vi "Application Status View.vi"(0 "Model in":refnum<class "Model.lvclass">) -> ()   [LabVIEW 2016, in "M1M3SupportEUI_Views.lvlib"]
uses:
  M1M3SupportEUI_Views.lvlib
  Model/Model.lvclass
  M1M3 Support Events/M1M3 Support Events.lvclass/M1M3 Support Events.ctl
  M1M3 Support Events/M1M3 Support Events.lvclass
panel:
  out "Force Magnitude":sgl format="%_8f"
  out "Mx":sgl format="%_8f"
  out "My":sgl format="%_8f"
  out "Mz":sgl format="%_8f"
  out "Fz":sgl format="%_8f"
  out "Fy":sgl format="%_8f"
  out "Fx":sgl format="%_8f"
  out "FA Force Warning Status":string
  out "FA Warning Status":string
  out "Summary State":string
  out "Interlock Status":string
  out "Detailed State":string
  # "Applied Forces Event Data"
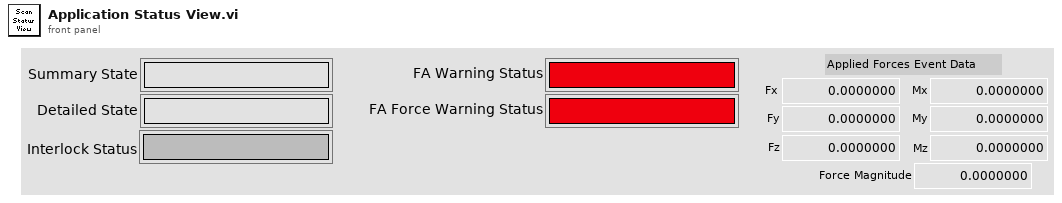
[diagram p1: front panel]
types:
  T1 = typedef "M1M3SupportEUI_TypeDefs.lvlib/M1M3 Support Events.ctl" = cluster{"Inclinometer  Data":refnum<user-event>, "IMS Data":refnum<user-event>, "SAL Connected":refnum<user-event>, "Accelerometer Data":refnum<user-event>, "OuterLoop Data":refnum<user-event>, "ErrorCode Event":refnum<user-event>, "InterlockStatus Event":refnum<user-event>, "InterlockWarning Event":refnum<user-event>, "Gyro Data":refnum<user-event>, "HP Actuator Info Event":refnum<user-event>, " FA Info Event":refnum<user-event>, "HP Monitor Info Event":refnum<user-event>, "FA Data":refnum<user-event>, "HP Actuator data":refnum<user-event>, "HP Monitor data":refnum<user-event>, "Air Supply Status Event":refnum<user-event>, "Air Supply Warning Event":refnum<user-event>, "Power Data":refnum<user-event>, "PID Data":refnum<user-event>, "PID Info Event":refnum<user-event>, "Power Status Event":refnum<user-event>, "Power Supply Status Event":refnum<user-event>, "Power Warning Event":refnum<user-event>, "Summary State Event":refnum<user-event>, "Detailed State Event":refnum<user-event>, "FA Force Warning Event":refnum<user-event>, "FA Warning Event":refnum<user-event>, "FA State Event":refnum<user-event>, "Applied AberrationForces Event":refnum<user-event>, "Applied Acceleration Forcces Event":refnum<user-event>, "Applied Azimuth Forces Event":refnum<user-event>, "Applied Active Optic Forces Event":refnum<user-event>, "Applied Balance Forces Event":refnum<user-event>, "Applied Cylinder Forces Event":refnum<user-event>, "Applied Elevation Forces Event":refnum<user-event>, "Applied Forces Event":refnum<user-event>, "Applied Offset Forces Event":refnum<user-event>, "Applied Static Forces Event":refnum<user-event>, "Applied Thermal Forces Event":refnum<user-event>, "Applied Velocity Forces Event":refnum<user-event>, "Rejected Aberration Force Event":refnum<user-event>, "Rejected Acceleration Forces Event":refnum<user-event>, "Rejected Active Optic Forces Event":refnum<user-event>, "Rejected Azimuth Forces Event":refnum<user-event>, "Rejected Balance Forces Event":refnum<user-event>, "Rejected Cylinder Forces Event":refnum<user-event>, "Rejected Elevation Forces Event":refnum<user-event>, "Rejected Forces Event":refnum<user-event>, "Rejected Offset Forces Event":refnum<user-event>, "Rejected Static Forces Event":refnum<user-event>, "Rejected Thermal Forces Event":refnum<user-event>, "Rejected Velocity Forces Event":refnum<user-event>, "Command Rejection Event":refnum<user-event>, "Setting Verions Event":refnum<user-event>, "Settings Applied Event":refnum<user-event>}
  T2 = enum16{"", "DetailedState_DetailedStates_DisabledState", "DetailedState_DetailedStates_EnabledState", "DetailedState_DetailedStates_FaultState", "DetailedState_DetailedStates_OfflineState", "DetailedState_DetailedStates_StandbyState", "DetailedState_DetailedStates_ParkedState", "DetailedState_DetailedStates_RaisingState", "DetailedState_DetailedStates_ActiveState", "DetailedState_DetailedStates_LoweringState", "DetailedState_DetailedStates_EngineeringState", "DetailedState_DetailedStates_ParkedEngineeringState", "DetailedState_DetailedStates_RaisingEngineeringState", "DetailedState_DetailedStates_ActiveEngineeringState", "DetailedState_DetailedStates_LoweringEngineeringState", "DetailedState_DetailedStates_LoweringFaultState", "DetailedState_DetailedStates_ProfileHardpointCorrectionState"}
  T3 = enum16{"", "SummaryState_SummaryStates_DisabledState", "SummaryState_SummaryStates_EnabledState", "SummaryState_SummaryStates_FaultState", "SummaryState_SummaryStates_OfflineState", "SummaryState_SummaryStates_StandbyState"}
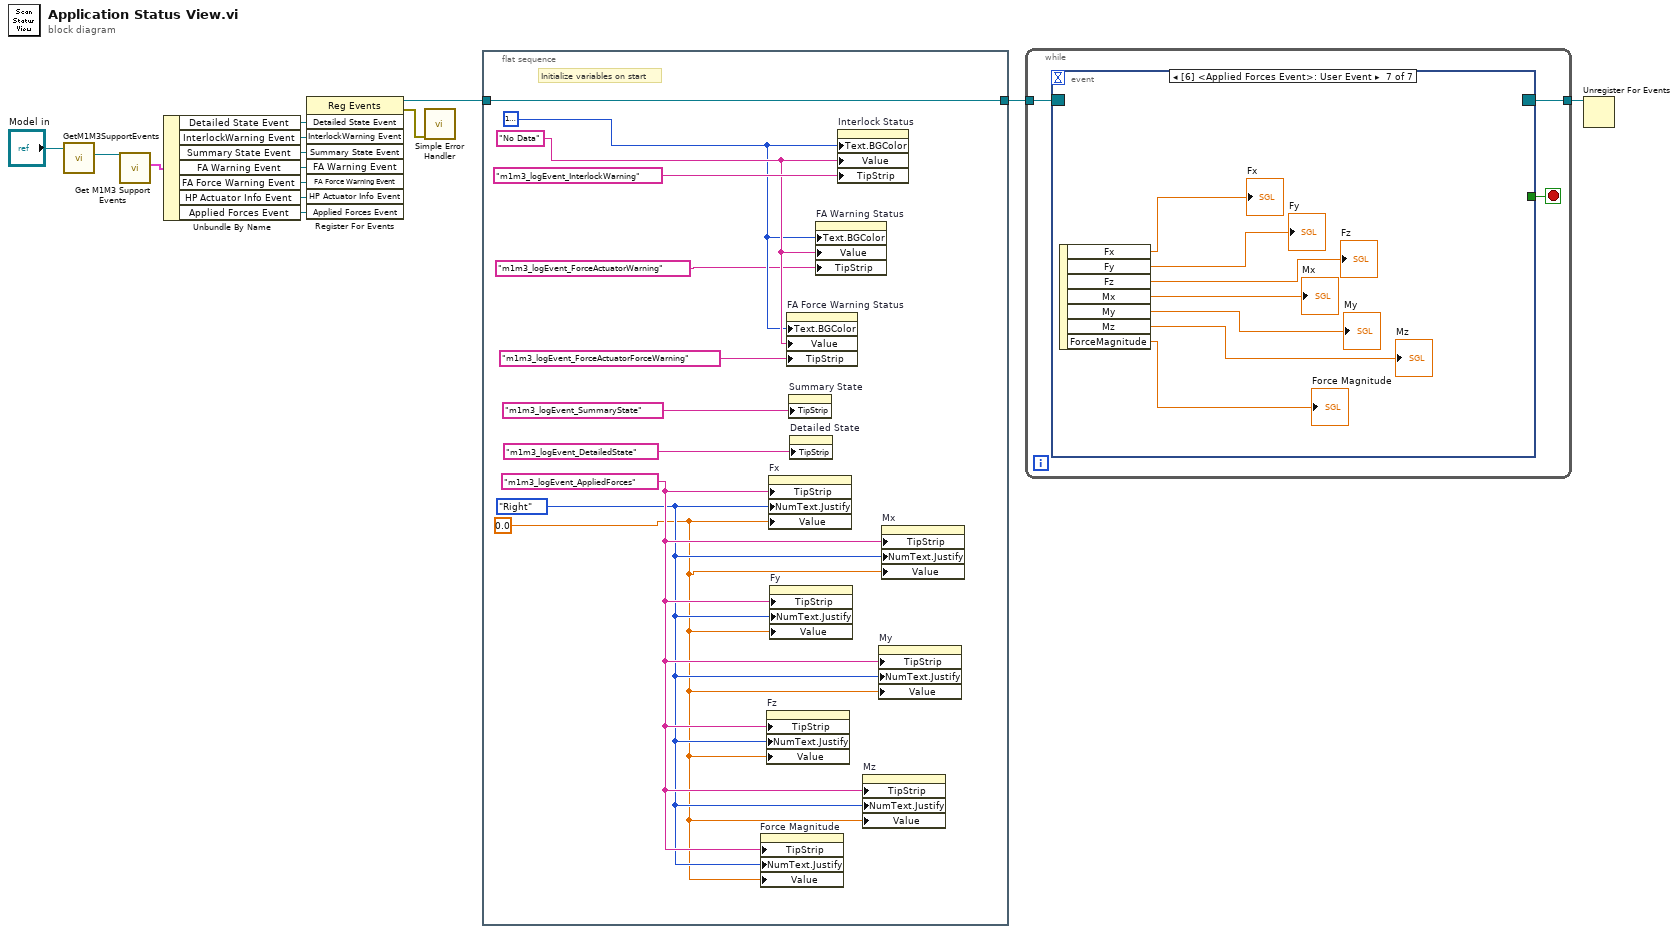
[diagram p0: block diagram]
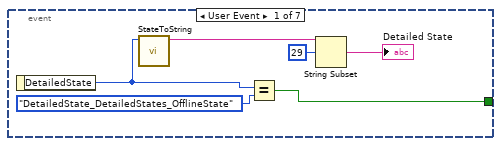
[diagram p2: hidden frame]
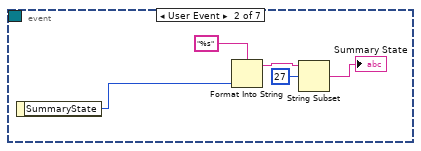
[diagram p3: hidden frame]
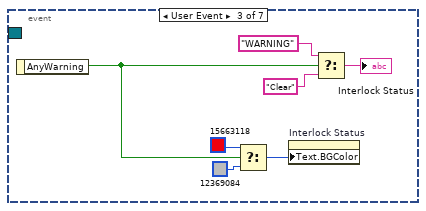
[diagram p4: hidden frame]
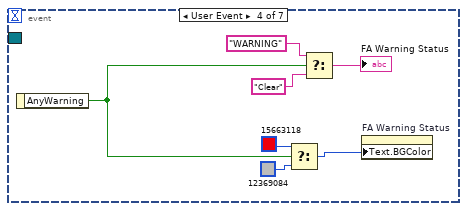
[diagram p5: hidden frame]
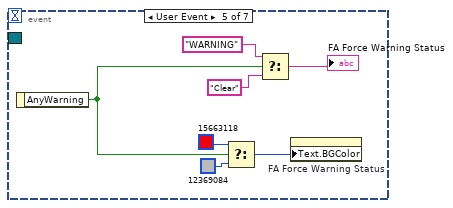
[diagram p6: hidden frame]
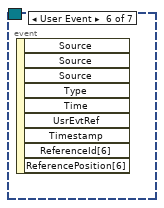
[diagram p7: hidden frame]
diagram:
  n1 = call "GetM1M3SupportEvents.vi"("Model in"="Model in") -> ("M1M3 Support Events out"=w9:refnum<class "M1M3 Support Events.lvclass">)  [unwired: 8 in, 2 out]
  n2 = call "Get M1M3 Support Events.vi"("M1M3 Support Events in"=w9) -> ("M1M3 Support Events"=w14:T1)  [unwired: 9 in, 1 out]
  n3 = Unbundle By Name(w14) -> ("Detailed State Event"=w13:refnum<user-event>, "InterlockWarning Event"=w8:refnum<user-event>, "Summary State Event"=w5:refnum<user-event>, "FA Warning Event"=w4:refnum<user-event>, "FA Force Warning Event"=w3:refnum<user-event>, "HP Actuator Info Event"=w2:refnum<user-event>, "Applied Forces Event"=w1:refnum<user-event>)
  n4 = register-events(w13, w8, w5, w4, w3, w2, w1) -> (reference out=w7:refnum<event-registration>, error out=w11:errorcluster)  [unwired: 2 in]
  n5 = call <vilib>:"Simple Error Handler.vi"("error in (no error)"=w11) -> ()  [unwired: 4 in, 5 out]
  n6 = flat-sequence {
    tunnel: w7 -> [w25]
    tunnel: [w25] -> w6
    frame #0 {
      w15 = 0.0 ("Fx")
      w16 = enum16{"Left", "Center", "Right"}."Right" ("Numeric Text.Justification")
      w17 = "m1m3_logEvent_AppliedForces" ("Tip Strip")
      w20 = u32 16777238
      w21 = "No Data"
      # "Initialize variables on start"
      n7 = property on="Force Magnitude" class="DigNum (strict)"("TipStrip"=w17, "NumText.Justify"=w16, "Value"=w15) -> ()  [unwired: 2 in, 2 out]
      n8 = property on="Fz" class="DigNum (strict)"("TipStrip"=w17, "NumText.Justify"=w16, "Value"=w15) -> ()  [unwired: 2 in, 2 out]
      n9 = property on="Fx" class="DigNum (strict)"("TipStrip"=w17, "NumText.Justify"=w16, "Value"=w15) -> ()  [unwired: 2 in, 2 out]
      n10 = property on="Fy" class="DigNum (strict)"("TipStrip"=w17, "NumText.Justify"=w16, "Value"=w15) -> ()  [unwired: 2 in, 2 out]
      n11 = property on="FA Force Warning Status" class="Str"("Text.BGColor"=w20, "Value"=w21, "TipStrip"="m1m3_logEvent_ForceActuatorForceWarning" ("Tip Strip")) -> ()  [unwired: 2 in, 2 out]
      n12 = property on="Summary State" class="Str"("TipStrip"="m1m3_logEvent_SummaryState" ("Tip Strip")) -> ()  [unwired: 2 in, 2 out]
      n13 = property on="Detailed State" class="Str"("TipStrip"="m1m3_logEvent_DetailedState" ("Tip Strip")) -> ()  [unwired: 2 in, 2 out]
      n14 = property on="FA Warning Status" class="Str"("Text.BGColor"=w20, "Value"=w21, "TipStrip"="m1m3_logEvent_ForceActuatorWarning" ("Tip Strip")) -> ()  [unwired: 2 in, 2 out]
      n15 = property on="Interlock Status" class="Str"("Text.BGColor"=w20, "Value"=w21, "TipStrip"="m1m3_logEvent_InterlockWarning" ("Tip Strip")) -> ()  [unwired: 2 in, 2 out]
      n16 = property on="Mz" class="DigNum (strict)"("TipStrip"=w17, "NumText.Justify"=w16, "Value"=w15) -> ()  [unwired: 2 in, 2 out]
      n17 = property on="My" class="DigNum (strict)"("TipStrip"=w17, "NumText.Justify"=w16, "Value"=w15) -> ()  [unwired: 2 in, 2 out]
      n18 = property on="Mx" class="DigNum (strict)"("TipStrip"=w17, "NumText.Justify"=w16, "Value"=w15) -> ()  [unwired: 2 in, 2 out]
    }
  }
  n19 = while {
    tunnel: w6 -> [w28]
    tunnel: [w27] -> w12
    stop <- w26 stop-if-true
    n20 = event shown="[6] <Applied Forces Event>: User Event" {
      selector: w28 -> [_ _ _ _ _ _ _]
      dyn-events: [_ _ _ _ _ _ _] -> w27
      timeout: _ -> [_ _ _ _ _ _ _]
      tunnel: [w34 _ _ _ _ _ _] -> w26
      event User Event {
        n21 = event-data() -> ("DetailedState"=w33:T2)  [unwired: 1 in]
        n22 = call "StateToString.vi"("DetailedState"=w33) -> ("State Type String"=w29:string)  [unwired: 10 in]
        n23 = Equal?(x=w33, y=T2."DetailedState_DetailedStates_OfflineState") -> (x = y?=w34:bool)
        n24 = String Subset(string=w29, offset (0)=29) -> (substring=→"Detailed State":string)  [unwired: 1 in]
      }
      event User Event {
        n25 = event-data() -> ("SummaryState"=w38:T3)  [unwired: 1 in]
        n26 = Format Into String(format string="%s", w38) -> (resulting string=w36:string)  [unwired: 2 in, 1 out]
        n27 = String Subset(string=w36, offset (0)=27) -> (substring=→"Summary State":string)  [unwired: 1 in]
      }
      event User Event {
        n28 = event-data() -> ("AnyWarning"=w40:bool)  [unwired: 1 in]
        n29 = Select(t=u32 15663118, s=w40, f=u32 12369084) -> (s? t:f=w41:u32)
        n30 = property on="Interlock Status" class="Str"("Text.BGColor"=w41) -> ()  [unwired: 2 in, 2 out]
        n31 = Select(t="WARNING", s=w40, f="Clear") -> (s? t:f=→"Interlock Status":string)
      }
      event User Event {
        n32 = event-data() -> ("AnyWarning"=w49:bool)  [unwired: 1 in]
        n33 = Select(t=u32 15663118, s=w49, f=u32 12369084) -> (s? t:f=w47:u32)
        n34 = Select(t="WARNING", s=w49, f="Clear") -> (s? t:f=→"FA Warning Status":string)
        n35 = property on="FA Warning Status" class="Str"("Text.BGColor"=w47) -> ()  [unwired: 2 in, 2 out]
      }
      event User Event {
        n36 = event-data() -> ("AnyWarning"=w56:bool)  [unwired: 1 in]
        n37 = Select(t=u32 15663118, s=w56, f=u32 12369084) -> (s? t:f=w54:u32)
        n38 = Select(t="WARNING", s=w56, f="Clear") -> (s? t:f=→"FA Force Warning Status":string)
        n39 = property on="FA Force Warning Status" class="Str"("Text.BGColor"=w54) -> ()  [unwired: 2 in, 2 out]
      }
      event User Event {
        n40 = event-data() -> ()  [unwired: 1 in, 9 out]
      }
      event User Event {
        n41 = event-data() -> ("Fx"=→"Fx":sgl, "Fy"=→"Fy":sgl, "Fz"=→"Fz":sgl, "Mx"=→"Mx":sgl, "My"=→"My":sgl, "Mz"=→"Mz":sgl, "ForceMagnitude"=→"Force Magnitude":sgl)  [unwired: 1 in]
      }
    }
  }
  n42 = Unregister For Events(event registration refnum=w12) -> ()  [unwired: 1 in, 1 out]
